vi "Write Plugin Address.vi"(8 "error in (no error)":errorcluster, 10 "Plugin Address":string, 11 "MeasurementSMO in":refnum<class "MeasurementSMO.lvclass">) -> (0 "error out":errorcluster, 3 "MeasurementSMO out":refnum<class "MeasurementSMO.lvclass">)   [LabVIEW 2019, in "MeasurementSMO.lvclass"]
uses:
  MeasurementSMO.lvclass
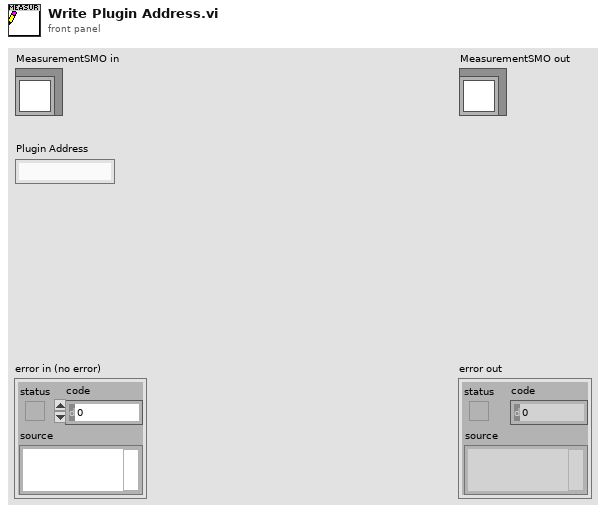
[diagram p1: front panel]
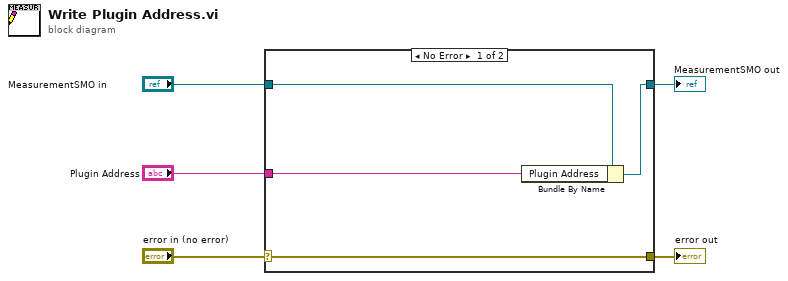
[diagram p0: block diagram]
diagram:
  n1 = case shown="No Error" "error in (no error)" {
    selector: "error in (no error)" -> [w9 w10]
    tunnel: [w9 w10] -> w4
    tunnel: [w7 w11] -> w2
    tunnel: "MeasurementSMO in" -> [w8 w11]
    tunnel: "Plugin Address" -> [w6 _]
    frame No Error {
      n2 = Bundle By Name(cluster=w8, "Plugin Address"=w6) -> (w7:refnum<class "MeasurementSMO.lvclass">)
    }
    frame Error {
    }
  }
  "error out" <- w4
  "MeasurementSMO out" <- w2
